vi "Enumerate API.vi"(8 "error in (no error)":errorcluster, 11 "Child Class in":refnum<class "Instrument.lvclass">) -> (0 "error out":errorcluster, 2 "Methods":string[](array[string]), 3 "Child Class out":refnum<class "Instrument.lvclass">)   [LabVIEW 2017, in "Instrument.lvlib" / "Instrument.lvclass"]
uses:
  Instrument.lvclass
  <vilib>/TSS/ACRObat Test Framework/Classes/Base Objects/Acrobat Base Object/Acrobat Base Object/Acrobat Base Object.lvclass
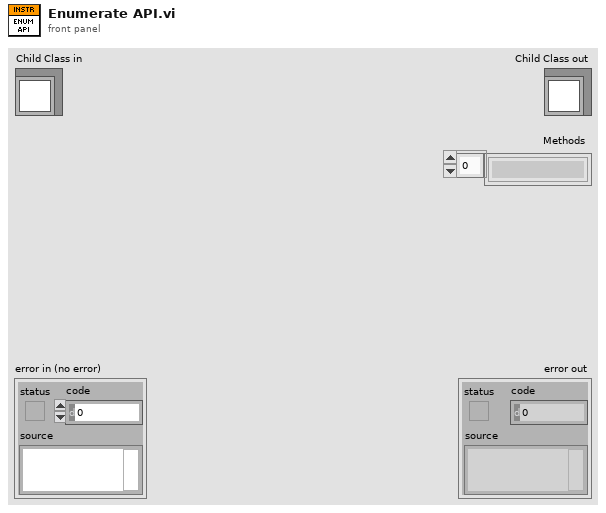
[diagram p1: front panel]
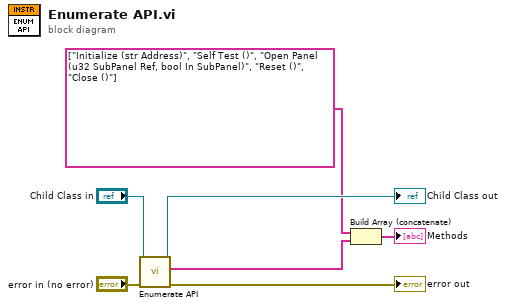
[diagram p0: block diagram]
diagram:
  n1 = call-parent "Enumerate API.vi"("error in (no error)"="error in (no error)", "Child Class in"="Child Class in") -> ("error out"=→"error out":errorcluster, "Methods"=w6:string[], "Child Class out"=→"Child Class out":refnum<class "Instrument.lvclass">)  [unwired: 7 in]
  n2 = Build Array (concatenate)(string[] ["Initialize (str Address)", "Self Test ()", "Open Panel (u32 SubPanel Ref, bool In SubPanel)", "Reset ()", "Close ()"] ("array"), w6) -> (→"Methods":string[])
